vi "Abandon Changes Prompt.vi"(11 "Entity Editor":refnum<class "Entity Editor.lvclass">) -> (2 "Confirmed?":bool)   [LabVIEW 2020, in "Conditum-Tools.lvlib" / "Entity Editor.lvclass"]
uses:
  Entity Editor.lvclass
  Entity Editor.lvclass/Entity Editor.ctl
panel:
  in  "Cancel":bool
  in  "OK":bool
  # "You have unsaved changes!\nDo you want to continue?"
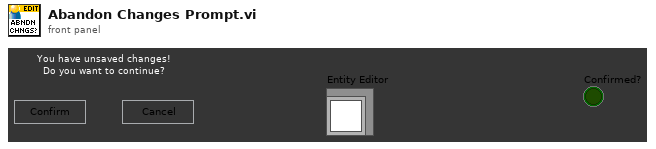
[diagram p1: front panel]
types:
  T1 = enum32{"Invalid", "Standard", "Closed", "Hidden", "Minimized", "Maximized"}
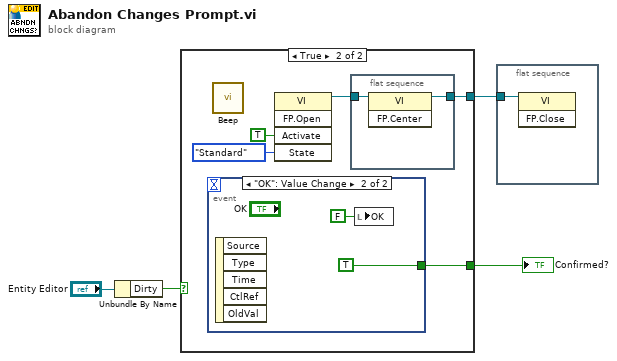
[diagram p0: block diagram]
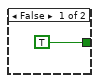
[diagram p2: hidden frame]
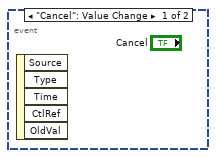
[diagram p3: hidden frame]
diagram:
  n1 = Unbundle By Name("Entity Editor") -> ("Dirty"=w2:bool)
  n2 = case shown="True" w2 {
    tunnel: [TRUE w10] -> w4
    tunnel: [_ w6] -> w1
    frame False {
    }
    frame True {
      n3 = event shown="[1] \"OK\": Value Change" {
        selector: _ -> [_ _]
        dyn-events: _ -> [_ _]
        timeout: _ -> [_ _]
        tunnel: [_ TRUE] -> w10
        event "Cancel": Value Change {
          n4 = event-data() -> ()  [unwired: 1 in, 5 out]
        }
        event "OK": Value Change {
          n5 = event-data() -> ()  [unwired: 1 in, 5 out]
          n6 = local write "OK"(FALSE ("OK")) -> ()
        }
      }
      n7 = call <vilib>:"Beep.vi"() -> ()  [unwired: 12 in]
      n8 = invoke class="VI" method="FP.Open"("Activate"=TRUE ("Activate?"), "State"=T1."Standard") -> (reference out=w9:refnum<vi>)  [unwired: 3 in, 4 out]
      n9 = flat-sequence {
        tunnel: w9 -> [w12]
        tunnel: [w11] -> w6
        frame #0 {
          n10 = invoke class="VI" method="FP.Center"(reference=w12) -> (reference out=w11:refnum<vi>)  [unwired: 2 in, 2 out]
        }
      }
    }
  }
  "Confirmed?" <- w4
  n11 = flat-sequence {
    tunnel: w1 -> [w15]
    frame #0 {
      n12 = invoke class="VI" method="FP.Close"(reference=w15) -> ()  [unwired: 2 in, 3 out]
    }
  }
